vi "Gen Ball Trajectory.vi"(11 "Robot Velocities":T1) -> (2 "Auto Positions":cluster{"x":dbl, "y":dbl, dbl}[](array[cluster]), 3 "Auto Velocities":cluster{"x out":dbl, "y out":dbl, "Omega":dbl}[](array[cluster]))   [LabVIEW 2025]
uses:
  swerve-template/Type Definitions/Data/Robot Velocities.ctl
  <vilib>/Analysis/coordinate.llb/2D Cartesian Coordinate Rotation (Scalar).vi
  Framework/Robot Global Data.vi
  <vilib>/Analysis/NI_AALPro.lvlib
panel:
  out "Array":cluster{"x":dbl, "y":dbl, dbl}[](array[cluster])
  out "Traj Vel Points":T2(array[cluster])
  out "Traj Pos Points":cluster{"x":dbl, "y":dbl, "th":dbl}[](array[cluster])
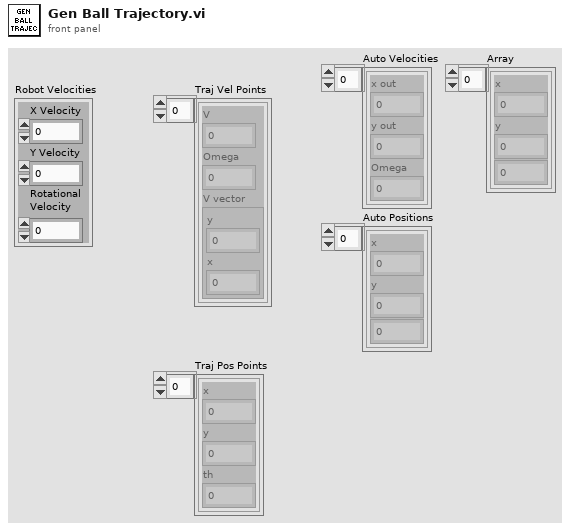
[diagram p1: front panel]
types:
  T1 = typedef "Robot Velocities.ctl" = cluster{"X Velocity":dbl, "Y Velocity":dbl, "Rotational \nVelocity":dbl}
  T2 = cluster{"V":dbl, "Omega":dbl, "V vector":cluster{"y":dbl, "x":dbl}}[]
  T3 = cluster{cluster{"X":dbl, "Y":dbl, dbl}, cluster{dbl, dbl, dbl}}[]
  T4 = typedef "Segment Type.ctl" = enum16{"Accel Straight", "Const Straight", "Blend", "Circle", "Bezier"}
  T5 = cluster{"Segment Name":string, "Type":T4, "Traj Pos Points":cluster{"x":dbl, "y":dbl, "th":dbl}[], "Traj Vel Points":cluster{"V":dbl, "Omega":dbl, "V vector":cluster{"y":dbl, "x":dbl}}[], "Accel Index":i32, "Decel Index":i32}[]
  T6 = cluster{"Segment Name":string, "Type":T4, "Traj Pos Points":cluster{"x":dbl, "y":dbl, "th":dbl}[], "Traj Vel Points":cluster{"V":dbl, "Omega":dbl, "V vector":cluster{"y":dbl, "x":dbl}}[], "Accel Index":i32, "Decel Index":i32}
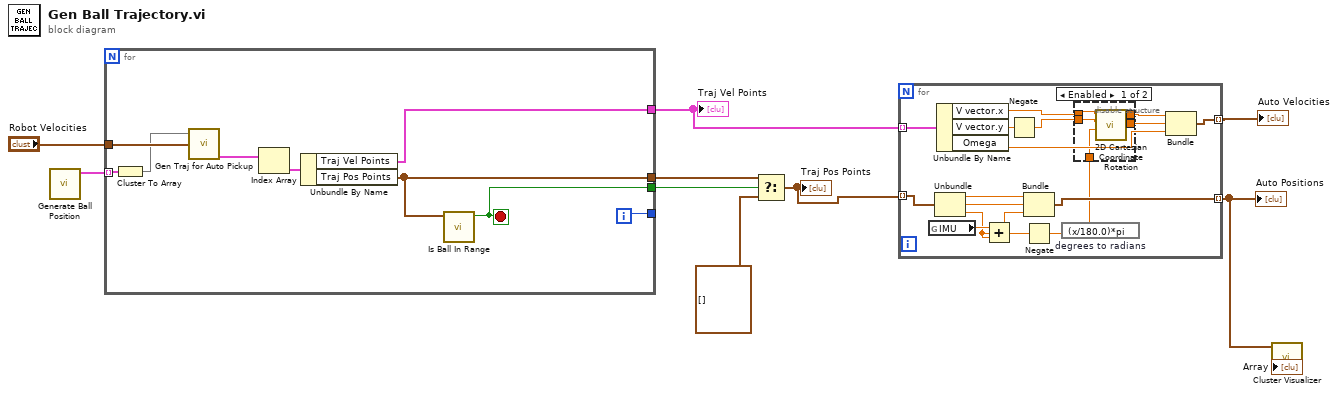
[diagram p0: block diagram]
diagram:
  n1 = call "Generate Ball Position.vi"() -> ("Array"=w1:T3)  [unwired: 11 in]
  n2 = for {
    tunnel: "Robot Velocities" -> [w16]
    tunnel: [w15] -> w8
    tunnel: [w14] -> w5
    tunnel: w1 -> [w12] mode=indexing
    tunnel: [w13] -> _
    tunnel: [w10] -> w3
    i -> [w13]
    stop <- w10 stop-if-true
    n3 = Cluster To Array(cluster=w12) -> (array=w11:cluster{"X":dbl, "Y":dbl, dbl}[])
    n4 = call "Gen Traj for Auto Pickup.vi"("Path Positions"=w11, "Robot Velocities"=w16) -> ("Trajectory Data Out"=w18:T5)  [unwired: 2 in, 2 out]
    n5 = Index Array(array=w18) -> (element=w17:T6)  [unwired: 1 in]
    n6 = Unbundle By Name(w17) -> ("Traj Vel Points"=w14:T2, "Traj Pos Points"=w15:cluster{"x":dbl, "y":dbl, "th":dbl}[])
    n7 = call "Is Ball In Range.vi"("Traj Pos Points in"=w15) -> ("logical AND"=w10:bool)  [unwired: 10 in]
  }
  "Traj Vel Points" <- w5
  n8 = Select(t=w8, s=w3, f=cluster{"x":dbl, "y":dbl, "th":dbl}[] []) -> (s? t:f=w6:cluster{"x":dbl, "y":dbl, "th":dbl}[])
  "Traj Pos Points" <- w6
  n9 = for {
    tunnel: w5 -> [w35] mode=indexing
    tunnel: w6 -> [w32] mode=indexing
    tunnel: [w31] -> w2 mode=indexing
    tunnel: [w25] -> w4 mode=indexing
    n10 = global read "Robot Global Data.vi" "IMU"() -> (w30:dbl)
    n11 = Unbundle(w32) -> ("x"=w33:dbl, "y"=w34:dbl, "th"=w22:dbl)
    n12 = Unbundle By Name(w35) -> ("V vector.x"=w20:dbl, "V vector.y"=w29:dbl, "Omega"=w26:dbl)
    n13 = Add(x=w30, y=w22) -> (x+y=w23:dbl)
    n14 = Negate(x=w29) -> (-x=w28:dbl)
    n15 = Bundle("x"=w33, "y"=w34, w23) -> (w31:cluster{"x":dbl, "y":dbl, dbl})  [unwired: 1 in]
    n16 = Negate(x=w22) -> (-x=w24:dbl)
    n17 = expression code="(x/180.0)*pi" "degrees to radians"(w24) -> (w21:dbl)
    n18 = disable-structure shown="Enabled" {
      disable-tunnel: w20 -> [w40 w42]
      disable-tunnel: w28 -> [w39 w41]
      disable-tunnel: [w38 w42] -> w19
      disable-tunnel: [w37 w41] -> w27
      disable-tunnel: w21 -> [w36 _]
      frame Enabled {
        n19 = call-poly <vilib>:"2D Cartesian Coordinate Rotation.vi"("theta"=w36, "y"=w39, "x"=w40) -> ("y out"=w37:dbl, "x out"=w38:dbl)  [unwired: 6 in, 1 out]
      }
      frame Disabled {
      }
    }
    n20 = Bundle("x out"=w19, "y out"=w27, "Omega"=w26) -> (w25:cluster{"x out":dbl, "y out":dbl, "Omega":dbl})  [unwired: 1 in]
  }
  "Auto Velocities" <- w4
  "Auto Positions" <- w2
  n21 = call "Cluster Visualizer.vi"("Array in"=w2) -> ()  [unwired: 11 in]
